vi "计算修正传输波数k.vi"(9 "f":dbl[](array[numeric]), 10 "c0":dbl, 11 "dia_tube(m)":dbl) -> (3 "k":cdb[](array[numeric]))   [LabVIEW 2018]
panel:
  out "RE":cluster{"X":dbl, "Y":dbl}[](graph)
  out "IM":cluster{"X":dbl, "Y":dbl}[](graph)
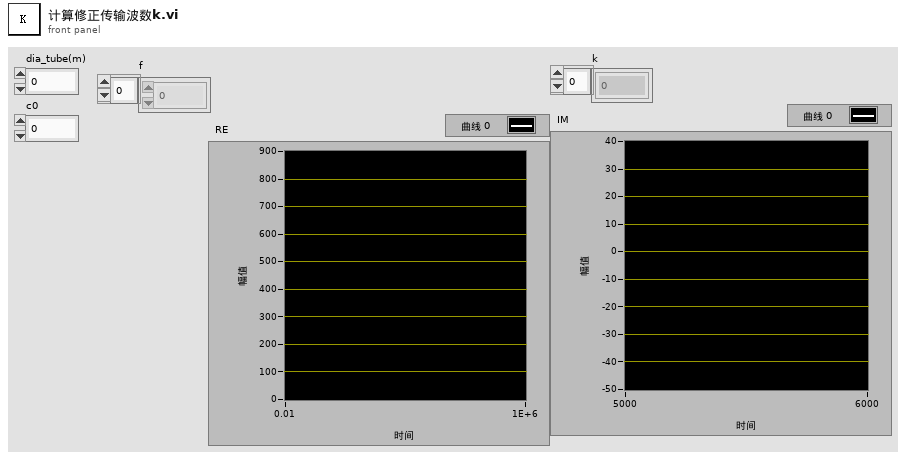
[diagram p1: front panel]
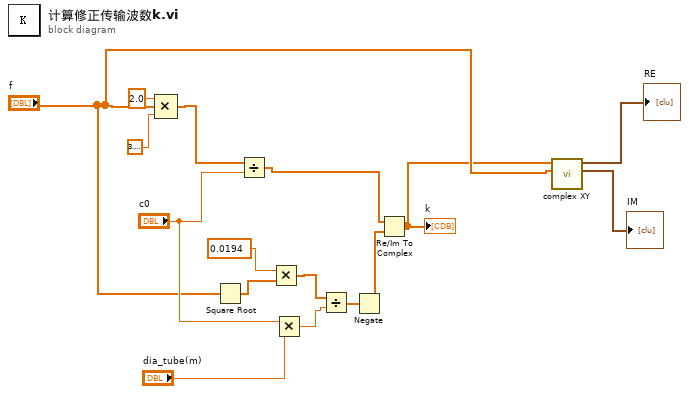
[diagram p0: block diagram]
diagram:
  n1 = Compound Arithmetic op=MULTIPLY(2.0 ("值"), "f", 3.141592653589793) -> (w14:dbl[])
  n2 = Square Root(x="f") -> (sqrt(x)=w9:dbl[])
  n3 = Divide(x=w14, y="c0") -> (x/y=w13:dbl[])
  n4 = Multiply(x=0.0194, y=w9) -> (x*y=w12:dbl[])
  n5 = Multiply(x="c0", y="dia_tube(m)") -> (x*y=w11:dbl)
  n6 = Divide(x=w12, y=w11) -> (x/y=w6:dbl[])
  n7 = Negate(x=w6) -> (-x=w5:dbl[])
  n8 = Re/Im To Complex(1:w5, 2:w13) -> (0:w3:cdb[])
  "k" <- w3
  n9 = call "complex XY.vi"("f"="f", "数组"=w3) -> ("IM"=→"IM":cluster{"X":dbl, "Y":dbl}[], "RE"=→"RE":cluster{"X":dbl, "Y":dbl}[])  [unwired: 8 in]
